vi "Setup.vi"(8 "error in (no error)":errorcluster, 11 "LUnit Setup Error In":refnum<class "LUnit Setup Error.lvclass">) -> (0 "error out":errorcluster, 3 "LUnit Setup Error Out":refnum<class "LUnit Setup Error.lvclass">)   [LabVIEW 2020, in "LUnit Setup Error.lvclass"]
uses:
  LUnit Setup Error.lvclass
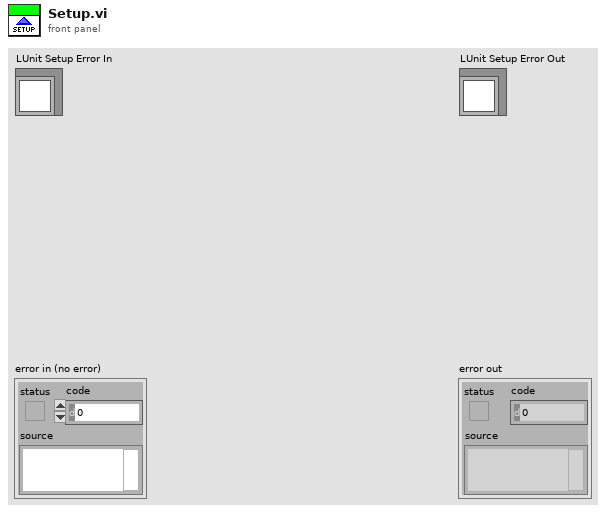
[diagram p1: front panel]
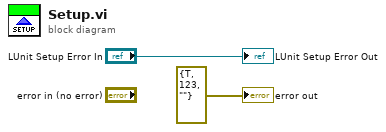
[diagram p0: block diagram]
diagram:
  "error out" <- errorcluster {"status"=TRUE, "code"=123, "source"=""} ("error out")
  "LUnit Setup Error Out" <- "LUnit Setup Error In"
